vi "02 - Calling C Cpp and CLI.vi"   [LabVIEW 2021]
panel:
  # "RUN VI to launch needed example project\n(finds example in current LabVIEW version)\nCtl+R"
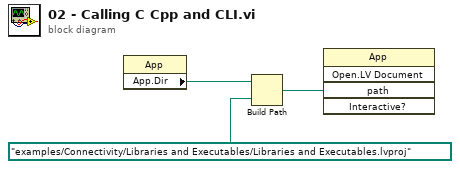
[diagram p0: block diagram]
diagram:
  n1 = property class="App"() -> ("App.Dir"=w1:path)  [unwired: 2 in, 2 out]
  n2 = Build Path(base path=w1, name or relative path=path "examples/Connectivity/Libraries and Executables/Libraries and Executables.lvproj") -> (appended path=w2:path)
  n3 = invoke class="App" method="Open.LV Document"("path"=w2) -> ()  [unwired: 4 in, 5 out]
